vi "Set.vi"(10 "Value":dbl, 11 "Double in":refnum<class "Double.lvclass">) -> (3 "Double out":refnum<class "Double.lvclass">)   [LabVIEW 2020, in "Conditu2.lvlib" / "Columns.lvlib" / "Double.lvclass"]
uses:
  Double.lvclass
  Double.lvclass/Double.ctl
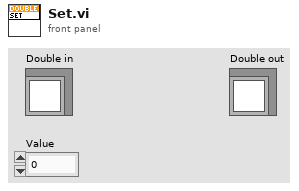
[diagram p1: front panel]
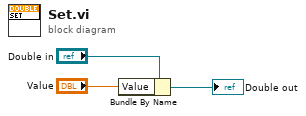
[diagram p0: block diagram]
diagram:
  n1 = Bundle By Name(cluster="Double in", "Value"="Value") -> (→"Double out":refnum<class "Double.lvclass">)
